vi "Select Higher than Threshold.vi"(0 "Function In":cluster{"Z":dbl[], "Score":sgl[]}) -> (1 "Function Out":cluster{"Z":dbl[], "Score":sgl[]}, 2 "Indexes":i32[](array[numeric]))   [LabVIEW 2014]
panel:
  in  "Threshold":sgl
  # "LICENSED MATERIALS – PROPERTY OF IBM\nCopyright IBM Corp. 2016,\nALL RIGHTS RESERVED"
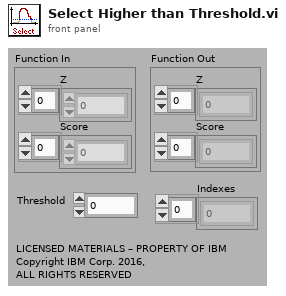
[diagram p1: front panel]
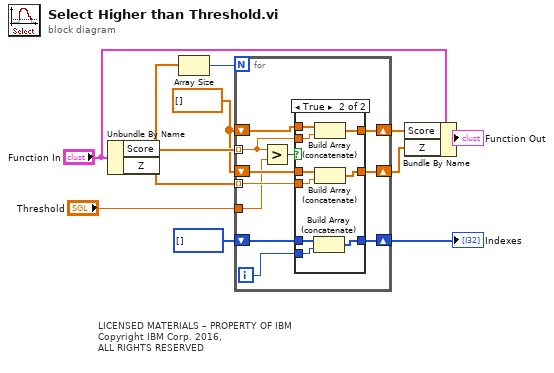
[diagram p0: block diagram]
diagram:
  w6 = dbl[] [] ("Array")
  # "LICENSED MATERIALS – PROPERTY OF IBM\nCopyright IBM Corp. 2016,\nALL RIGHTS RESERVED"
  n1 = Unbundle By Name("Function In") -> ("Score"=w8:sgl[], "Z"=w7:dbl[])
  n2 = Array Size(array=w8) -> (size(s)=w9:i32)
  n3 = for {
    N: w9 -> [_]
    tunnel: w8 -> [w13] mode=indexing
    shift-right: [w20] -> w5
    shift-left: w6 -> [w21]
    tunnel: w7 -> [w17] mode=indexing
    shift-right: [w19] -> w4
    shift-left: w6 -> [w18]
    shift-right: [w14] -> w2
    shift-left: i32[] [] ("Array") -> [w15]
    tunnel: "Threshold" -> [w12]
    i -> [w16]
    n4 = Greater?(x=w13, y=w12) -> (0:w22:bool)
    n5 = case shown="True" w22 {
      tunnel: w21 -> [w25 w34]
      tunnel: w13 -> [_ w33]
      tunnel: [w25 w32] -> w20
      tunnel: [w24 w31] -> w19
      tunnel: w18 -> [w24 w29]
      tunnel: w17 -> [_ w30]
      tunnel: w16 -> [_ w28]
      tunnel: w15 -> [w23 w27]
      tunnel: [w23 w26] -> w14
      frame False {
      }
      frame True {
        n6 = Build Array (concatenate)(w27, w28) -> (w26:i32[])
        n7 = Build Array (concatenate)(w34, w33) -> (w32:dbl[])
        n8 = Build Array (concatenate)(w29, w30) -> (w31:dbl[])
      }
    }
  }
  "Indexes" <- w2
  n9 = Bundle By Name(cluster="Function In", "Score"=w5, "Z"=w4) -> (→"Function Out":cluster{"Z":dbl[], "Score":sgl[]})
